vi "Max Time.vi"(1 "Max Time":dbl, 2 "Reset?":bool) -> (0 "Finished?":bool)   [LabVIEW 2016]
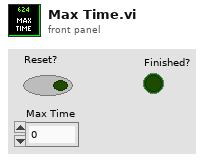
[diagram p1: front panel]
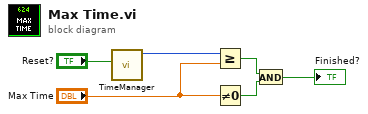
[diagram p0: block diagram]
diagram:
  n1 = call "TimeManager.vi"("Reset?"="Reset?") -> ("Time Since Reset"=w5:u32)  [unwired: 9 in, 1 out]
  n2 = Greater Or Equal?(x=w5, y="Max Time") -> (x >= y?=w2:bool)
  n3 = Not Equal To 0?(x="Max Time") -> (x != 0?=w3:bool)
  n4 = And(x=w2, y=w3) -> (x .and. y?=→"Finished?":bool)
